vi "Main FPGA 5-axis for XYZ.vi"() -> ()   [LabVIEW 2014]
uses:
  <vilib>/Motion/MotorControl/_s/nism.interpretControlRegister.stateTransition.ctl
  <vilib>/Platform/TimedLoop/XDataNode/timing_clust.ctl
  <vilib>/Platform/TimedLoop/XDataNode/nitl_modes.ctl
  <vilib>/Platform/TimedLoop/XDataNode/wakeup.ctl
  <vilib>/Motion/MotorControl/_s/nism.digitalInputs.portA.ctl
  <vilib>/rvi/Emulation/niFpgaGetClockAttributes.vi
  <vilib>/rvi/Emulation/niFpgaSctlEmulationGetInTimedLoop.vi
  <vilib>/rvi/Emulation/niFpgaEmulationReportErrorSimple.vi
  Global FPGA.vi
  <vilib>/Motion/MotorControl/_s/nism.interpretControlRegister.indexed.vi
  <vilib>/rvi/Emulation/niFpgaProcessEmulError.vi
  <vilib>/Motion/MotorControl/_s/nism.mdo.read.positionLoopSyncData.vi
  <vilib>/Motion/MotorControl/_s/nism.mdo.read.splineData.vi
  <vilib>/Motion/MotorControl/_s/nism.generateStatusRegister.indexed.vi
  <vilib>/rvi/eio/common/nirviEmuTemplateMethod_errors.vi
  <vilib>/rvi/Emulation/niFpgaCriticalErrorInLSC.vi
  <vilib>/Motion/MotorControl/_s/nism.splineInterpolation.fxp.3.index.vi
  <vilib>/Motion/MotorControl/_s/nism.mdo.handler.indexed.vi
  <vilib>/Motion/MotorControl/_s/nism.digitalFilter.indexed.vi
  <vilib>/Motion/MotorControl/_s/nism.interpretDIOControl.portA.multiple.vi
  <vilib>/Motion/MotorControl/_s/nism.generateDIOStatus.portA.indexed.2.vi
  <vilib>/Motion/SoftMotion/Synchronization/nism.rioScan.generateSyncScan.vi
  <vilib>/eio/EIONode/EIONode.xnode
  <vilib>/Platform/TimedLoop/XDataNode/XDataNode.xnode
  <vilib>/Motion/MotorControl/NI_SoftMotion_MotorControlIP.lvlib
  <vilib>/Platform/TimedLoop/XDataNode/XDNodeRunTimeDep.lvlib
  <vilib>/Motion/SoftMotion/Synchronization/NI_SoftMotion_Synchronization.lvlib
panel:
  in  "Mod3/DIO31":bool
  in  "Mod3/DIO30":bool
  in  "Mod3/DIO29":bool
  in  "Mod3/DIO28":bool
  in  "Fwd 5":bool
  in  "Fwd 4":bool
  in  "Rev 5":bool
  in  "Rev 4":bool
  in  "Home 5":bool
  in  "Home 4":bool
  out "Home Limits":bool[](array[boolean])
  out "Fwd Limits":bool[](array[boolean])
  out "Rev Limits":bool[](array[boolean])
  out "Axis Positions":fxp<+/-,64,32>[](array[numeric])
  in  "STEP or CW? (T=STEP)":bool
  out "Drive Enable":bool[](array[boolean])
  in  "Enable Watchdog":bool
  in  "Pet Watchdog":bool
  in  "Watchdog Timeout Period (ticks)":u64=40000000 format="%.0p"
  out "Watchdog Timed Out?":bool
  out "Time Since Last Pet":u64
  in  "Enable value":bool
  in  "Drive Enable override?":bool
  out "State":T1=enum."Start --> Initializing" caption="state transition"
  in  "Sync Value":bool
  in  "Sync Enable override?":bool
  in  "Invert direction?":bool
  out "Sync is Fault":bool
  out "Sync is Locked":bool
  in  "minimum pulse":u16=40
  # "Synchronization Loop"
  # "Control Status Loop"
  # "Notes: \n1. This VI provides the communication interface between the NI SoftMotion Engine and the LabVIEW FPGA Module. You must compile this VI for a specific FPGA target before use. After compiling, run the VI before running any of the Express VI examples. For information on moving this example to another FPGA target, refer to ni.com/info and enter info code fpgaex.\n\n2. Only use the Reset Axis button if you are unable to communicate with the axis by any other means. This button resets the device state machine and other VIs to a known state. After resetting the axis, switch the NI Scan Engine from Active Mode to Configuration Mode, then back to Active Mode, before attempting to enable the axis."
  # "(These two buttons \nare for testing\npurposes.)"
  # "(These two buttons \nare for testing\npurposes.)"
  # "Step/Direction Loop"
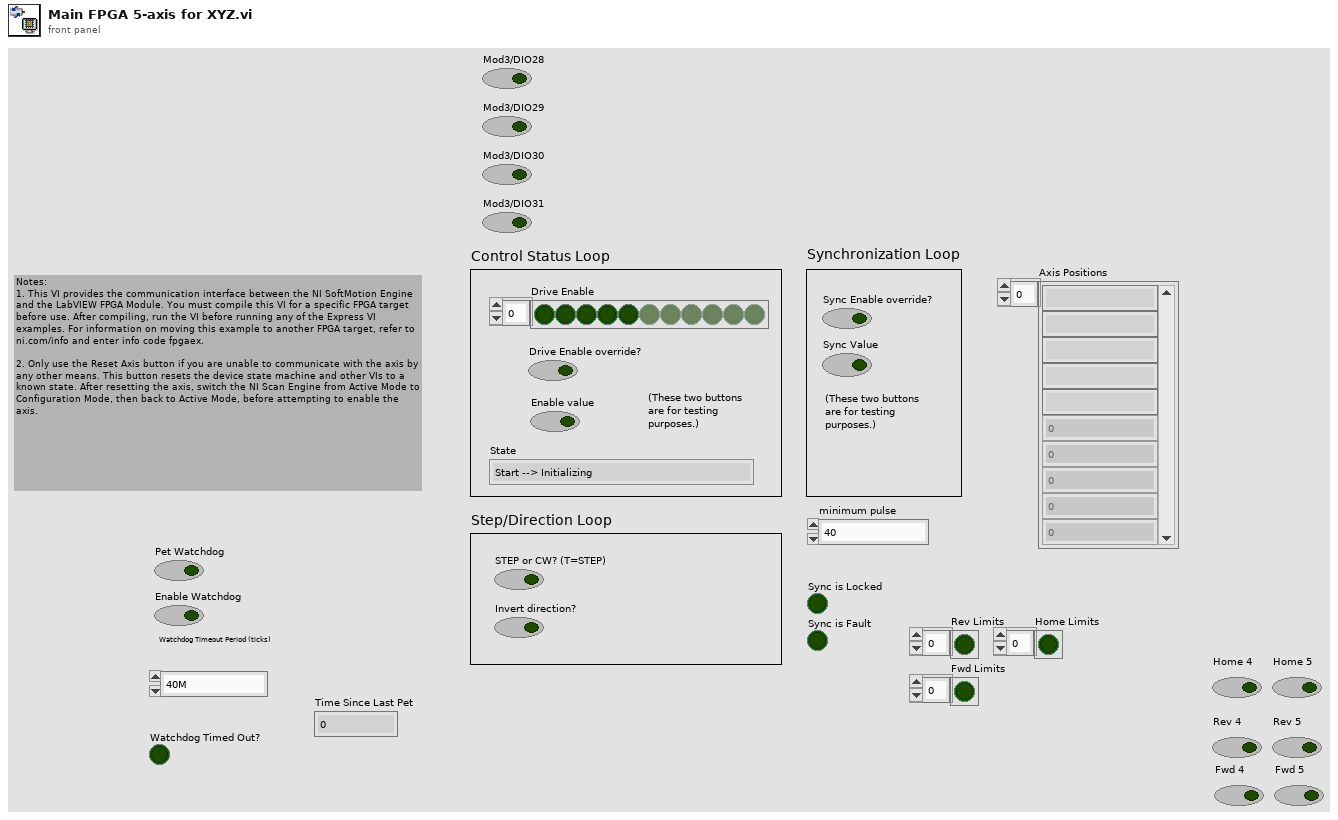
[diagram p1: front panel]
types:
  T1 = typedef "NI_SoftMotion_MotorControlIP.lvlib/nism.interpretControlRegister.stateTransition.ctl" = enum8{"Invalid", "Start --> Initializing", "Initializing --> Disabled", "Disabled --> Ready To Switch On", "Ready To Switch On --> Switched On", "Ready To Switch On --> Disable", "Switched On --> Operation Enable", "Switched On --> Ready To Switch On", "Switched On --> Disabled", "Operation Enable --> Switched On", "Operation Enable --> Ready To Switch On", "Operation Enable --> Disabled", "Fault --> Disabled", "Any --> Fault", "None"}
  T2 = typedef "NI_SoftMotion_Synchronization.lvlib/nism.softmotionScan.timerConfig.ctl" = cluster{"target period (clocks)":u16, "host period / target period":u16}
  T3 = typedef "NI_SoftMotion_MotorControlIP.lvlib/nism.mdo.splineData.ctl" = cluster{"spline type":T4, "traj per/spline per":u16, "spline per/traj per":fxp<+,32,0>}
  T4 = typedef "NI_SoftMotion_MotorControlIP.lvlib/nism.splineInterpolation.type.ctl" = u16
  T5 = typedef "XDNodeRunTimeDep.lvlib/timing_clust.ctl" = cluster{"Expected End [f-1]":u64, "Actual End [f-1]":u64, "Finished Late? [f-1]":bool, "Expected End [i-1]":u64, "Actual End [i-1]":u64, "Finished Late? [i-1]":bool, "Expected Start [i]":u64, "Actual Start [i]":u64, "Expected Start [f]":u64, "Actual Start [f]":u64, "Source Name":string, "Structure Name":string, "Period":i64, "Deadline":i64, "Offset":i64, "Start":i64, "Priority":i32, "Timeout":i32, "Mode":T6, "Wakeup Reason":T7, "Error":errorcluster, "Source Type":string, "Secondary Source Type":string, "Global End Time":u64, "Global Start Time":u64, "Frame Duration":u64, "Iteration Duration":u64, "Assigned CPU":i32, "I/O Scan Engine Mode":u32}
  T6 = typedef "XDNodeRunTimeDep.lvlib/nitl_modes.ctl" = enum32{"No Change", "Process missed periods, maintain original phase", "Discard missed periods, maintain original phase", "Process missed periods, ignore original phase", "Discard missed periods, ignore original phase"}
  T7 = typedef "XDNodeRunTimeDep.lvlib/wakeup.ctl" = enum32{"Normal", "Aborted", "Asynchronous wakeup", "Timing source error", "Timed loop error", "Timeout"}
  T8 = typedef "NI_SoftMotion_Synchronization.lvlib/nism.softmotionScan.timerControl.ctl" = cluster{"sm scan":bool, "sm scan count":u32, "sm scan enabled":bool}
  T9 = typedef "NI_SoftMotion_MotorControlIP.lvlib/nism.digitalInputs.portA.ctl" = cluster{"reverse limit":bool, "forward limit":bool, "home switch":bool, "digital input 0":bool, "digital input 1":bool, "digital input 2":bool, "digital input 3":bool}
  T10 = typedef "NI_SoftMotion_MotorControlIP.lvlib/nism.dio.portA.config.2.ctl" = cluster{"digital filter (us)":u16[], "safe state":T11[]}
  T11 = typedef "nism.safeStates.ctl" = enum8{"Low", "High", "No Change"}
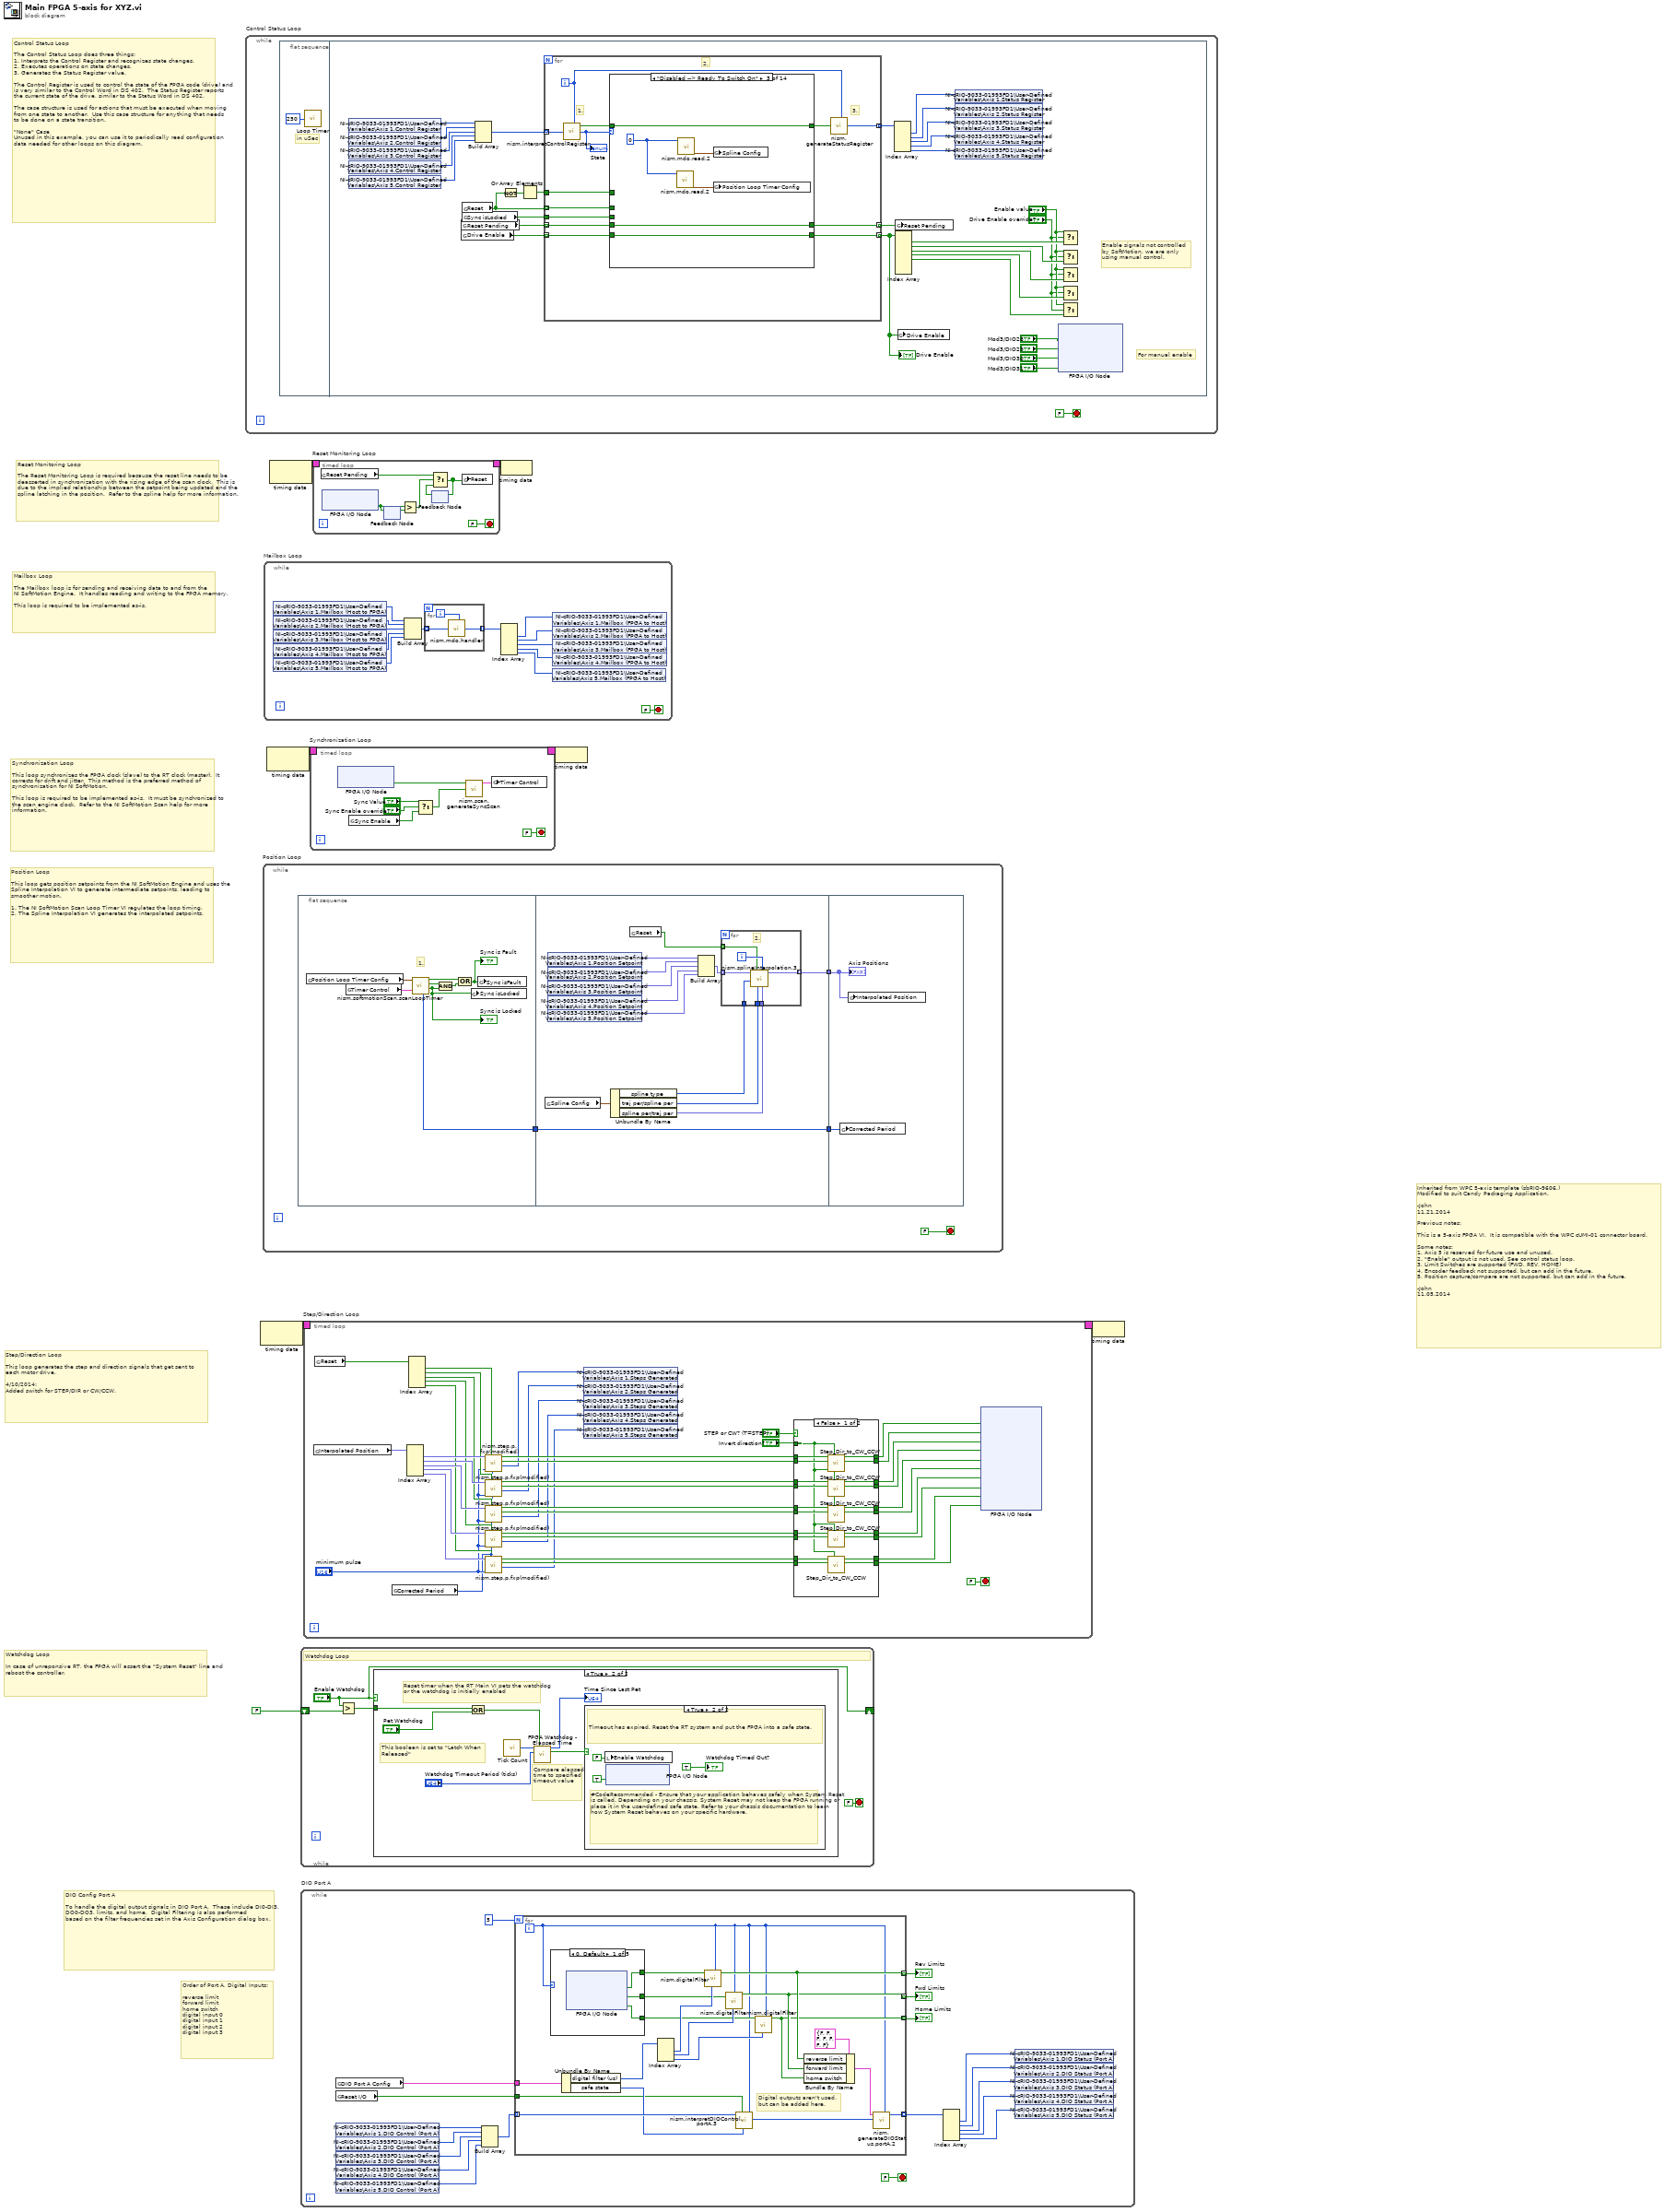
[diagram p0: block diagram]
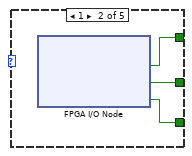
[diagram p2: hidden frame]
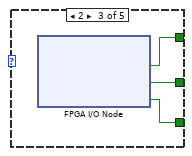
[diagram p3: hidden frame]
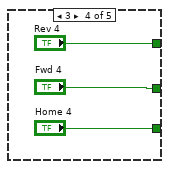
[diagram p4: hidden frame]
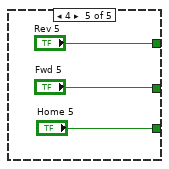
[diagram p5: hidden frame]
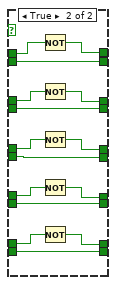
[diagram p9: hidden frame]
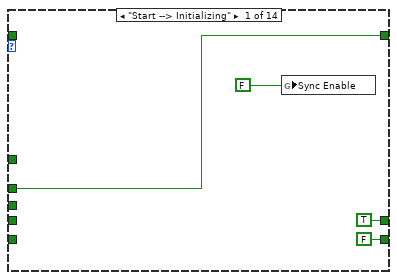
[diagram p10: hidden frame]
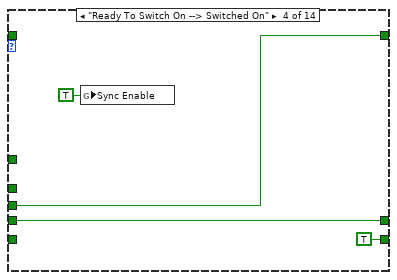
[diagram p12: hidden frame]
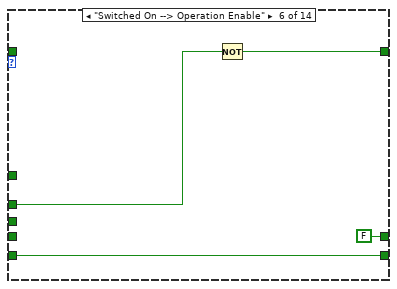
[diagram p14: hidden frame]
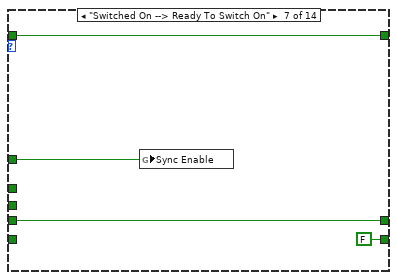
[diagram p15: hidden frame]
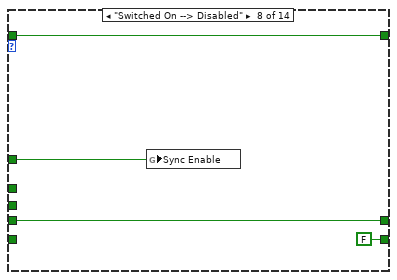
[diagram p16: hidden frame]
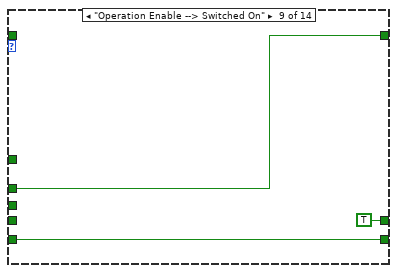
[diagram p17: hidden frame]
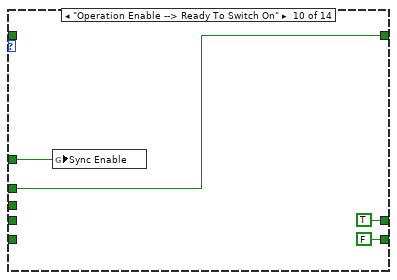
[diagram p18: hidden frame]
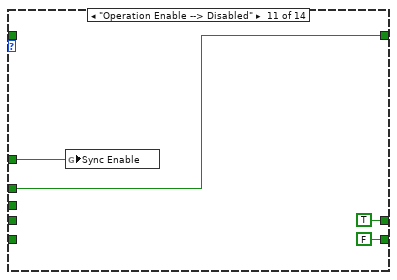
[diagram p19: hidden frame]
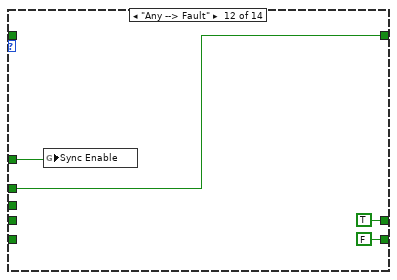
[diagram p20: hidden frame]
diagram:
  # "Inherited from WPC 5-axis template (sbRIO-9606.)\nModified to suit Candy Packaging Application.\n\n-John\n11.21.2014\n\nPrevious notes:\n\nThis is a 5-axis FPGA VI.  It is compatible with the WPC cUMI-01 connector board.\n\nSome notes:\n1. Axis 5 is reserved for future use and unused.\n2. \"Enable\" output is not used. See control status loop.\n3. Limit Switches are supported (FWD, REV, HOME)\n4. Encoder feedback not supported, but can add in the future.\n5. Position capture/compare are not supported, but can add in the future.\n\n-John\n11.05.2014"
  # "DIO Config Port A\n\nTo handle the digital output signals in DIO Port A.  These include DI0-DI3, DO0-DO3, limits, and home.  Digital Filtering is also performed\nbased on the filter frequencies set in the Axis Configuration dialog box."
  # "Order of Port A, Digital Inputs:\n\nreverse limit\nforward limit\nhome switch\ndigital input 0\ndigital input 1\ndigital input 2\ndigital input 3"
  # "Watchdog Loop\n\nIn case of unreponsive RT, the FPGA will assert the \"System Reset\" line and reboot the controller."
  # "Step/Direction Loop\n\nThis loop generates the step and direction signals that get sent to \neach motor drive.\n\n4/10/2014:\nAdded switch for STEP/DIR or CW/CCW."
  # "Position Loop\n\nThis loop gets position setpoints from the NI SoftMotion Engine and uses the Spline Interpolation VI to generate intermediate setpoints, leading to smoother motion.\n\n1. The NI SoftMotion Scan Loop Timer VI regulates the loop timing. \n2. The Spline Interpolation VI generates the interpolated setpoints."
  # "Synchronization Loop\n\nThis loop synchronizes the FPGA clock (slave) to the RT clock (master).  It corrects for drift and jitter.  This method is the preferred method of synchronization for NI SoftMotion.\n\nThis loop is required to be implemented as-is.  It must be synchronized to the scan engine clock.  Refer to the NI SoftMotion Scan help for more information."
  # "Mailbox Loop\n\nThe Mailbox loop is for sending and receiving data to and from the \nNI SoftMotion Engine.  It handles reading and writing to the FPGA memory.\n\nThis loop is required to be implemented as-is."
  # "Reset Monitoring Loop\n\nThe Reset Monitoring Loop is required because the reset line needs to be deasserted in synchronization with the rising edge of the scan clock.  This is due to the implied relationship between the setpoint being updated and the spline latching in the position.  Refer to the spline help for more information."
  # "Control Status Loop\n\nThe Control Status Loop does three things:\n1. Interprets the Control Register and recognizes state changes.\n2. Executes operations on state changes.\n3. Generates the Status Register value.\n\nThe Control Register is used to control the state of the FPGA code (drive) and is very similar to the Control Word in DS 402.  The Status Register reports the current state of the drive, similar to the Status Word in DS 402.\n\nThe case structure is used for actions that must be executed when moving from one state to another.  Use this case structure for anything that needs to be done on a state transition.\n\n\"None\" Case\nUnused in this example, you can use it to periodically read configuration data needed for other loops on this diagram."
  n1 = while "Control Status Loop" {
    stop <- FALSE stop-if-true
    n2 = flat-sequence {
      frame #0 {
        # "in uSec"
        n3 = call "Loop Timer"("Count(uSec)"=u32 250) -> ()  [unwired: 1 out]
      }
      frame #1 {
        # "For manual enable"
        # "Enable signals not controlled\nby SoftMotion, we are only\nusing manual control."
        n4 = shared-variable "NI-cRIO-9033-01993FD1\\User-Defined Variables\\Axis 1.Control Register"() -> (w30:u32)  [unwired: 1 in, 1 out]
        n5 = shared-variable "NI-cRIO-9033-01993FD1\\User-Defined Variables\\Axis 2.Control Register"() -> (w29:u32)  [unwired: 1 in, 1 out]
        n6 = shared-variable "NI-cRIO-9033-01993FD1\\User-Defined Variables\\Axis 3.Control Register"() -> (w28:u32)  [unwired: 1 in, 1 out]
        n7 = shared-variable "NI-cRIO-9033-01993FD1\\User-Defined Variables\\Axis 4.Control Register"() -> (w27:u32)  [unwired: 1 in, 1 out]
        n8 = shared-variable "NI-cRIO-9033-01993FD1\\User-Defined Variables\\Axis 5.Control Register"() -> (w26:u32)  [unwired: 1 in, 1 out]
        n9 = global read "Global FPGA.vi" "Reset Pending"() -> (w34:bool[])
        n10 = global read "Global FPGA.vi" "Drive Enable"() -> (w33:bool[])
        n11 = global read "Global FPGA.vi" "Reset"() -> (w35:bool[])
        n12 = global read "Global FPGA.vi" "Sync isLocked"() -> (w40:bool)
        n13 = Build Array(w30, w29, w28, w27, w26) -> (w39:u32[])
        n14 = Not(x=w35) -> (.not. x?=w37:bool[])
        n15 = Or Array Elements(Boolean array=w37) -> (logical OR=w36:bool)
        n16 = for {
          tunnel: w35 -> [w48] mode=indexing
          tunnel: w40 -> [w47]
          tunnel: w39 -> [w49] mode=indexing
          tunnel: [w46] -> w31 mode=indexing
          tunnel: [w45] -> w38 mode=indexing
          tunnel: [w44] -> w32 mode=indexing
          tunnel: w36 -> [w43]
          tunnel: w34 -> [w42] mode=indexing
          tunnel: w33 -> [w41] mode=indexing
          i -> [w50]
          # "3."
          # "2."
          # "1."
          n17 = call-poly <vilib>:"nism.interpretControlRegister.vi"("control register"=w49, "axis index"=w50) -> ("transition occurred"=w51:bool, "state transition"=w52:T1)  [unwired: 6 in]
          "State" <- w52
          n18 = case shown="\"Disabled --> Ready To Switch On\"" w52 {
            tunnel: w51 -> [_ w60 w66 _ w73 _ w81 w85 _ _ _ _ w105 _]
            tunnel: [w57 w60 w66 w68 w73 w77 w81 w85 w87 w90 w94 w98 w104 _] -> w53
            tunnel: w48 -> [w57 _ _ _ _ w76 _ _ w87 w90 w94 w98 _ _]
            tunnel: w47 -> [_ _ _ w68 _ _ _ _ _ _ _ _ _ _]
            tunnel: [TRUE ("Write.Reset Pending") w59 w63 w67 w72 FALSE ("Write.Reset Pending") w78 w82 TRUE ("Write.Reset Pending") TRUE ("Write.Reset Pending") TRUE ("Write.Reset Pending") TRUE ("Write.Reset Pending") w102 w107] -> w45
            tunnel: [FALSE ("Write.Drive Enable") w58 w62 TRUE ("Write.Drive Enable") w71 w74 FALSE ("Write.Drive Enable") FALSE ("Write.Drive Enable") w86 FALSE ("Write.Drive Enable") FALSE ("Write.Drive Enable") FALSE ("Write.Drive Enable") w101 w106] -> w44
            tunnel: w43 -> [_ _ _ _ _ _ w79 w83 _ w89 w93 w97 w103 _]
            tunnel: w42 -> [_ w59 w63 w67 w72 _ w78 w82 _ _ _ _ w102 w107]
            tunnel: w41 -> [_ w58 w62 _ w71 w74 _ _ w86 _ _ _ w101 w106]
            frame "Start --> Initializing" {
              n19 = global write "Global FPGA.vi" "Sync Enable"(FALSE ("Sync Enable")) -> ()
            }
            frame "Initializing --> Disabled" {
            }
            frame "Disabled --> Ready To Switch On" {
              w61 = 0 ("axis index")
              n20 = call-poly <vilib>:"nism.mdo.read.2.vi"("axis index"=w61) -> ("position loop sync"=w64:T2)  [unwired: 10 in]
              n21 = call-poly <vilib>:"nism.mdo.read.2.vi"("axis index"=w61) -> ("spline"=w65:T3)  [unwired: 10 in]
              n22 = global write "Global FPGA.vi" "Spline Config"(w65) -> ()
              n23 = global write "Global FPGA.vi" "Position Loop Timer Config"(w64) -> ()
            }
            frame "Ready To Switch On --> Switched On" {
              n24 = global write "Global FPGA.vi" "Sync Enable"(TRUE ("Sync Enable")) -> ()
            }
            frame "Ready To Switch On --> Disable" {
            }
            frame "Switched On --> Operation Enable" {
              n25 = Not(x=w76) -> (.not. x?=w77:bool)
            }
            frame "Switched On --> Ready To Switch On" {
              n26 = global write "Global FPGA.vi" "Sync Enable"(w79) -> ()
            }
            frame "Switched On --> Disabled" {
              n27 = global write "Global FPGA.vi" "Sync Enable"(w83) -> ()
            }
            frame "Operation Enable --> Switched On" {
            }
            frame "Operation Enable --> Ready To Switch On" {
              n28 = global write "Global FPGA.vi" "Sync Enable"(w89) -> ()
            }
            frame "Operation Enable --> Disabled" {
              n29 = global write "Global FPGA.vi" "Sync Enable"(w93) -> ()
            }
            frame "Any --> Fault" {
              n30 = global write "Global FPGA.vi" "Sync Enable"(w97) -> ()
            }
            frame "Fault --> Disabled" {
              # "wait one cycle for clear faults to have taken effect"
              n31 = global write "Global FPGA.vi" "Sync Enable"(w103) -> ()
              n32 = Not(x=w105) -> (.not. x?=w104:bool)
            }
            frame "None", Default {
            }
          }
          n33 = call-poly <vilib>:"nism.generateStatusRegister.vi"("transition success"=w53, "axis index"=w50) -> ("status register"=w46:u32)  [unwired: 7 in]
        }
        "Drive Enable" <- w32
        n34 = Index Array(array=w31) -> (element #1=w25:u32, element #2=w24:u32, element #3=w23:u32, element #4=w22:u32, element #5=w21:u32)  [unwired: 5 in]
        n35 = global write "Global FPGA.vi" "Reset Pending"(w38) -> ()
        n36 = Index Array(array=w32) -> (element #1=w20:bool, element #2=w19:bool, element #3=w18:bool, element #4=w17:bool, element #5=w16:bool)  [unwired: 8 in, 3 out]
        n37 = global write "Global FPGA.vi" "Drive Enable"(w32) -> ()
        n38 = shared-variable "NI-cRIO-9033-01993FD1\\User-Defined Variables\\Axis 1.Status Register"(w25) -> ()  [unwired: 1 in, 1 out]
        n39 = shared-variable "NI-cRIO-9033-01993FD1\\User-Defined Variables\\Axis 2.Status Register"(w24) -> ()  [unwired: 1 in, 1 out]
        n40 = shared-variable "NI-cRIO-9033-01993FD1\\User-Defined Variables\\Axis 3.Status Register"(w23) -> ()  [unwired: 1 in, 1 out]
        n41 = shared-variable "NI-cRIO-9033-01993FD1\\User-Defined Variables\\Axis 4.Status Register"(w22) -> ()  [unwired: 1 in, 1 out]
        n42 = shared-variable "NI-cRIO-9033-01993FD1\\User-Defined Variables\\Axis 5.Status Register"(w21) -> ()  [unwired: 1 in, 1 out]
        n43 = xnode "FPGA I/O Node"("Mod3/DIO28"="Mod3/DIO28", "Mod3/DIO29"="Mod3/DIO29", "Mod3/DIO30"="Mod3/DIO30", "Mod3/DIO31"="Mod3/DIO31") -> ()  [unwired: 4 in, 4 out]
        n44 = Select(t="Enable value", s="Drive Enable override?", f=w20) -> ()  [unwired: 1 out]
        n45 = Select(t="Enable value", s="Drive Enable override?", f=w19) -> ()  [unwired: 1 out]
        n46 = Select(t="Enable value", s="Drive Enable override?", f=w18) -> ()  [unwired: 1 out]
        n47 = Select(t="Enable value", s="Drive Enable override?", f=w17) -> ()  [unwired: 1 out]
        n48 = Select(t="Enable value", s="Drive Enable override?", f=w16) -> ()  [unwired: 1 out]
      }
    }
  }
  n49 = node-c288() -> (w7:T5)  [unwired: 1 in]
  n50 = while "Position Loop" {
    stop <- FALSE stop-if-true
    n51 = flat-sequence {
      tunnel: [w112] -> w108
      tunnel: [w126] -> w110
      tunnel: [w125] -> w109
      tunnel: w108 -> [w125]
      tunnel: w110 -> [w140]
      tunnel: w109 -> [w141]
      frame #0 {
        # "1."
        n52 = global read "Global FPGA.vi" "Position Loop Timer Config"() -> (w114:T2)
        n53 = global read "Global FPGA.vi" "Timer Control"() -> (w113:T8)
        n54 = call <vilib>:"nism.softmotionScan.scanLoopTimer.vi"("timer control"=w113, "timer config"=w114) -> ("scan running?"=w116:bool, "finished late?"=w118:bool, "fault occurred?"=w119:bool, "corrected period"=w112:u16)  [unwired: 5 in, 1 out]
        "Sync is Locked" <- w116
        n55 = Compound Arithmetic op=AND(w118, w116) -> (w117:bool)
        n56 = Compound Arithmetic op=OR(w119, w117) -> (w115:bool)
        "Sync is Fault" <- w115
        n57 = global write "Global FPGA.vi" "Sync isLocked"(w116) -> ()
        n58 = global write "Global FPGA.vi" "Sync isFault"(w115) -> ()
      }
      frame #1 {
        n59 = global read "Global FPGA.vi" "Spline Config"() -> (w128:T3)
        n60 = shared-variable "NI-cRIO-9033-01993FD1\\User-Defined Variables\\Axis 1.Position Setpoint"() -> (w124:fxp<+/-,64,32>)  [unwired: 1 in, 1 out]
        n61 = shared-variable "NI-cRIO-9033-01993FD1\\User-Defined Variables\\Axis 2.Position Setpoint"() -> (w123:fxp<+/-,64,32>)  [unwired: 1 in, 1 out]
        n62 = shared-variable "NI-cRIO-9033-01993FD1\\User-Defined Variables\\Axis 3.Position Setpoint"() -> (w122:fxp<+/-,64,32>)  [unwired: 1 in, 1 out]
        n63 = shared-variable "NI-cRIO-9033-01993FD1\\User-Defined Variables\\Axis 4.Position Setpoint"() -> (w121:fxp<+/-,64,32>)  [unwired: 1 in, 1 out]
        n64 = shared-variable "NI-cRIO-9033-01993FD1\\User-Defined Variables\\Axis 5.Position Setpoint"() -> (w120:fxp<+/-,64,32>)  [unwired: 1 in, 1 out]
        n65 = Unbundle By Name(w128) -> ("spline type"=w132:T4, "traj per/spline per"=w131:u16, "spline per/traj per"=w130:fxp<+,32,0>)
        n66 = global read "Global FPGA.vi" "Reset"() -> (w127:bool[])
        n67 = Build Array(w124, w123, w122, w121, w120) -> (w129:fxp<+/-,64,32>[])
        n68 = for {
          tunnel: w132 -> [w139]
          tunnel: w131 -> [w138]
          tunnel: w130 -> [w137]
          tunnel: w127 -> [w134] mode=indexing
          tunnel: w129 -> [w136] mode=indexing
          tunnel: [w133] -> w126 mode=indexing
          i -> [w135]
          # "2."
          n69 = call-poly <vilib>:"nism.splineInterpolation.3.vi"("1 / calls per sample"=w137, "index"=w135, "calls per sample"=w138, "reset"=w134, "spline type"=w139, "x"=w136) -> ("xi"=w133:fxp<+/-,64,32>)  [unwired: 4 in, 1 out]
        }
      }
      frame #2 {
        n70 = global write "Global FPGA.vi" "Corrected Period"(w141) -> ()
        n71 = global write "Global FPGA.vi" "Interpolated Position"(w140) -> ()
        "Axis Positions" <- w140
      }
    }
  }
  n72 = while "Mailbox Loop" {
    stop <- FALSE stop-if-true
    n73 = shared-variable "NI-cRIO-9033-01993FD1\\User-Defined Variables\\Axis 1.Mailbox (Host to FPGA)"() -> (w151:u64)  [unwired: 1 in, 1 out]
    n74 = shared-variable "NI-cRIO-9033-01993FD1\\User-Defined Variables\\Axis 2.Mailbox (Host to FPGA)"() -> (w150:u64)  [unwired: 1 in, 1 out]
    n75 = shared-variable "NI-cRIO-9033-01993FD1\\User-Defined Variables\\Axis 3.Mailbox (Host to FPGA)"() -> (w149:u64)  [unwired: 1 in, 1 out]
    n76 = shared-variable "NI-cRIO-9033-01993FD1\\User-Defined Variables\\Axis 4.Mailbox (Host to FPGA)"() -> (w148:u64)  [unwired: 1 in, 1 out]
    n77 = shared-variable "NI-cRIO-9033-01993FD1\\User-Defined Variables\\Axis 5.Mailbox (Host to FPGA)"() -> (w147:u64)  [unwired: 1 in, 1 out]
    n78 = Build Array(w151, w150, w149, w148, w147) -> (w153:u64[])
    n79 = for {
      tunnel: w153 -> [w157] mode=indexing
      tunnel: [w156] -> w152 mode=indexing
      i -> [w155]
      n80 = call-poly <vilib>:"nism.mdo.handler.vi"("mbox (host to fpga)"=w157, "axis index"=w155) -> ("mbox (fpga to host)"=w156:u64)  [unwired: 7 in]
    }
    n81 = Index Array(array=w152) -> (element #1=w146:u64, element #2=w145:u64, element #3=w144:u64, element #4=w143:u64, element #5=w142:u64)  [unwired: 5 in]
    n82 = shared-variable "NI-cRIO-9033-01993FD1\\User-Defined Variables\\Axis 5.Mailbox (FPGA to Host)"(w142) -> ()  [unwired: 1 in, 1 out]
    n83 = shared-variable "NI-cRIO-9033-01993FD1\\User-Defined Variables\\Axis 1.Mailbox (FPGA to Host)"(w146) -> ()  [unwired: 1 in, 1 out]
    n84 = shared-variable "NI-cRIO-9033-01993FD1\\User-Defined Variables\\Axis 2.Mailbox (FPGA to Host)"(w145) -> ()  [unwired: 1 in, 1 out]
    n85 = shared-variable "NI-cRIO-9033-01993FD1\\User-Defined Variables\\Axis 3.Mailbox (FPGA to Host)"(w144) -> ()  [unwired: 1 in, 1 out]
    n86 = shared-variable "NI-cRIO-9033-01993FD1\\User-Defined Variables\\Axis 4.Mailbox (FPGA to Host)"(w143) -> ()  [unwired: 1 in, 1 out]
  }
  n87 = node-c288() -> (w5:T5)  [unwired: 1 in]
  n88 = node-c288() -> (w3:T5)  [unwired: 1 in]
  n89 = while "RT Watchdog Loop" {
    shift-right: ["Enable Watchdog"] -> _
    shift-left: FALSE ("Enable RT Watchdog") -> [w161]
    stop <- FALSE stop-if-true
    # "Watchdog Loop"
    n90 = Greater?(x="Enable Watchdog", y=w161) -> (0:w158:bool)
    n91 = case shown="True" "Enable Watchdog" {
      tunnel: w158 -> [_ w164]
      frame False {
        # "This loop has to be explicitly enabled from the RT Main VI.  This reduces the possiblity of an endless reboot cycle."
      }
      frame True {
        # "This boolean is set to \"Latch When Released\""
        # "Compare elapsed time to specified timeout value"
        # "Reset timer when the RT Main VI pets the watchdog or the watchdog is initially enabled"
        n92 = Or(x=w164, y="Pet Watchdog") -> (x .or. y?=w163:bool)
        n93 = call "Tick Count"() -> ("Tick Count(Ticks)"=w167:u32)
        n94 = call "FPGA Watchdog - Elapsed Time.vi"("Reset"=w163, "Timeout Period"="Watchdog Timeout Period (ticks)", "Current Time"=w167) -> ("Timeout"=w162:bool, "Elapsed Time"=→"Time Since Last Pet":u64)  [unwired: 7 in]
        n95 = case shown="True" w162 {
          frame False {
            # "Timeout has not expired."
          }
          frame True {
            # "#CodeRecommended - Ensure that your application behaves safely when System Reset is called. Depending on your chassis, System Reset may not keep the FPGA running or place it in the user-defined safe state. Refer to your chassis documentation to learn how System Reset behaves on your specific hardware."
            # "Timeout has expired. Reset the RT system and put the FPGA into a safe state."
            n96 = local write "Enable Watchdog"(FALSE ("Enable RT Watchdog")) -> ()
            n97 = xnode "FPGA I/O Node"("System Reset"=TRUE ("RT Reset on Watchdog Failure?")) -> ()  [unwired: 1 in, 1 out]
            "Watchdog Timed Out?" <- TRUE ("Watchdog Timed Out?")
          }
        }
      }
    }
  }
  n98 = while "DIO Port A" {
    stop <- FALSE stop-if-true
    n99 = global read "Global FPGA.vi" "DIO Port A Config"() -> (w189:T10)
    n100 = global read "Global FPGA.vi" "Reset I/O"() -> (w188:bool)
    n101 = shared-variable "NI-cRIO-9033-01993FD1\\User-Defined Variables\\Axis 1.DIO Control (Port A)"() -> (w186:u32)  [unwired: 1 in, 1 out]
    n102 = shared-variable "NI-cRIO-9033-01993FD1\\User-Defined Variables\\Axis 2.DIO Control (Port A)"() -> (w185:u32)  [unwired: 1 in, 1 out]
    n103 = shared-variable "NI-cRIO-9033-01993FD1\\User-Defined Variables\\Axis 3.DIO Control (Port A)"() -> (w184:u32)  [unwired: 1 in, 1 out]
    n104 = shared-variable "NI-cRIO-9033-01993FD1\\User-Defined Variables\\Axis 4.DIO Control (Port A)"() -> (w183:u32)  [unwired: 1 in, 1 out]
    n105 = shared-variable "NI-cRIO-9033-01993FD1\\User-Defined Variables\\Axis 5.DIO Control (Port A)"() -> (w182:u32)  [unwired: 1 in, 1 out]
    n106 = Build Array(w186, w185, w184, w183, w182) -> (w181:u32[])
    n107 = for {
      N: 5 -> [_]
      tunnel: [w209] -> w175 mode=indexing
      tunnel: w181 -> [w208] mode=indexing
      tunnel: w189 -> [w206]
      tunnel: w188 -> [w204]
      tunnel: [w196] -> w174 mode=indexing
      tunnel: [w195] -> w173 mode=indexing
      tunnel: [w194] -> w172 mode=indexing
      i -> [w193]
      # "Digital outputs aren't used,\nbut can be added here."
      n108 = case shown="0, Default" w193 {
        tunnel: [w212 w215 w218 "Rev 4" "Rev 5"] -> w199
        tunnel: [w210 w213 w216 "Home 4" "Home 5"] -> w198
        tunnel: [w211 w214 w217 "Fwd 4" "Fwd 5"] -> w197
        frame 0, Default {
          n109 = xnode "FPGA I/O Node"() -> ("Mod3/DIO0"=w212:bool, "Mod3/DIO1"=w211:bool, "Mod3/DIO2"=w210:bool)  [unwired: 3 in, 3 out]
        }
        frame 1 {
          n110 = xnode "FPGA I/O Node"() -> ("Mod3/DIO3"=w215:bool, "Mod3/DIO4"=w214:bool, "Mod3/DIO5"=w213:bool)  [unwired: 3 in, 3 out]
        }
        frame 2 {
          n111 = xnode "FPGA I/O Node"() -> ("Mod3/DIO6"=w218:bool, "Mod3/DIO7"=w217:bool, "Mod3/DIO8"=w216:bool)  [unwired: 3 in, 3 out]
        }
        frame 3 {
        }
        frame 4 {
        }
      }
      n112 = Unbundle By Name(w206) -> ("digital filter (us)"=w200:u16[], "safe state"=w205:T11[])
      n113 = Index Array(array=w200) -> (element #1=w201:u16, element #2=w202:u16, element #3=w203:u16)  [unwired: 3 in]
      n114 = call-poly <vilib>:"nism.digitalFilter.vi"("index"=w193, "filter value (us)"=w201, "input signal"=w199) -> ("output signal"=w196:bool)  [unwired: 8 in]
      n115 = call-poly <vilib>:"nism.digitalFilter.vi"("index"=w193, "filter value (us)"=w202, "input signal"=w197) -> ("output signal"=w195:bool)  [unwired: 8 in]
      n116 = call-poly <vilib>:"nism.interpretDIOControl.portA.3.vi"("index"=w193, "safe state"=w205, "reset"=w204, "dio control(port a)"=w208) -> ("reset latches"=w191:u8)  [unwired: 6 in, 1 out]
      n117 = call-poly <vilib>:"nism.digitalFilter.vi"("index"=w193, "filter value (us)"=w203, "input signal"=w198) -> ("output signal"=w194:bool)  [unwired: 8 in]
      n118 = Bundle By Name(cluster=T9 {"reverse limit"=FALSE, "forward limit"=FALSE, "home switch"=FALSE, "digital input 0"=FALSE, "digital input 1"=FALSE, "digital input 2"=FALSE, "digital input 3"=FALSE} ("$(driveInterface.digitalInputs.shortName)"), "reverse limit"=w196, "forward limit"=w195, "home switch"=w194) -> (w192:T9)
      n119 = call-poly <vilib>:"nism.generateDIOStatus.portA.2.vi"("index"=w193, "reset latches"=w191, "digital inputs"=w192) -> ("dio status(port a)"=w209:u32)  [unwired: 8 in]
    }
    "Rev Limits" <- w174
    "Fwd Limits" <- w173
    "Home Limits" <- w172
    n120 = Index Array(array=w175) -> (element #1=w180:u32, element #2=w179:u32, element #3=w178:u32, element #4=w177:u32, element #5=w176:u32)  [unwired: 5 in]
    n121 = shared-variable "NI-cRIO-9033-01993FD1\\User-Defined Variables\\Axis 1.DIO Status (Port A)"(w180) -> ()  [unwired: 1 in, 1 out]
    n122 = shared-variable "NI-cRIO-9033-01993FD1\\User-Defined Variables\\Axis 2.DIO Status (Port A)"(w179) -> ()  [unwired: 1 in, 1 out]
    n123 = shared-variable "NI-cRIO-9033-01993FD1\\User-Defined Variables\\Axis 3.DIO Status (Port A)"(w178) -> ()  [unwired: 1 in, 1 out]
    n124 = shared-variable "NI-cRIO-9033-01993FD1\\User-Defined Variables\\Axis 4.DIO Status (Port A)"(w177) -> ()  [unwired: 1 in, 1 out]
    n125 = shared-variable "NI-cRIO-9033-01993FD1\\User-Defined Variables\\Axis 5.DIO Status (Port A)"(w176) -> ()  [unwired: 1 in, 1 out]
  }
  n126 = timed-loop "Step/Direction Loop" {
    timing: w7 -> [_]
    timing-out: [_] -> w6
    stop <- FALSE stop-if-true
    n127 = global read "Global FPGA.vi" "Interpolated Position"() -> (w265:fxp<+/-,64,32>[])
    n128 = global read "Global FPGA.vi" "Reset"() -> (w259:bool[])
    n129 = global read "Global FPGA.vi" "Corrected Period"() -> (w235:u16)
    n130 = Index Array(array=w265) -> (element #1=w264:fxp<+/-,64,32>, element #2=w263:fxp<+/-,64,32>, element #3=w262:fxp<+/-,64,32>, element #4=w261:fxp<+/-,64,32>, element #5=w260:fxp<+/-,64,32>)  [unwired: 5 in]
    n131 = Index Array(array=w259) -> (element #1=w258:bool, element #2=w257:bool, element #3=w256:bool, element #4=w255:bool, element #5=w254:bool)  [unwired: 5 in]
    n132 = call "nism.step.p.fxp(modified).vi"("calls per sample"=w235, "reset"=w258, "minimum pulse"="minimum pulse", "position setpoint"=w264) -> ("steps generated"=w240:i32, "step"=w252:bool, "direction"=w253:bool)  [unwired: 4 in, 1 out]
    n133 = call "nism.step.p.fxp(modified).vi"("calls per sample"=w235, "reset"=w257, "minimum pulse"="minimum pulse", "position setpoint"=w263) -> ("steps generated"=w239:i32, "step"=w250:bool, "direction"=w251:bool)  [unwired: 4 in, 1 out]
    n134 = call "nism.step.p.fxp(modified).vi"("calls per sample"=w235, "reset"=w256, "minimum pulse"="minimum pulse", "position setpoint"=w262) -> ("steps generated"=w238:i32, "step"=w248:bool, "direction"=w249:bool)  [unwired: 4 in, 1 out]
    n135 = call "nism.step.p.fxp(modified).vi"("calls per sample"=w235, "reset"=w255, "minimum pulse"="minimum pulse", "position setpoint"=w261) -> ("steps generated"=w237:i32, "step"=w246:bool, "direction"=w247:bool)  [unwired: 4 in, 1 out]
    n136 = call "nism.step.p.fxp(modified).vi"("calls per sample"=w235, "reset"=w254, "minimum pulse"="minimum pulse", "position setpoint"=w260) -> ("steps generated"=w236:i32, "step"=w244:bool, "direction"=w245:bool)  [unwired: 4 in, 1 out]
    n137 = shared-variable "NI-cRIO-9033-01993FD1\\User-Defined Variables\\Axis 1.Steps Generated"(w240) -> ()  [unwired: 1 in, 1 out]
    n138 = shared-variable "NI-cRIO-9033-01993FD1\\User-Defined Variables\\Axis 2.Steps Generated"(w239) -> ()  [unwired: 1 in, 1 out]
    n139 = shared-variable "NI-cRIO-9033-01993FD1\\User-Defined Variables\\Axis 3.Steps Generated"(w238) -> ()  [unwired: 1 in, 1 out]
    n140 = shared-variable "NI-cRIO-9033-01993FD1\\User-Defined Variables\\Axis 4.Steps Generated"(w237) -> ()  [unwired: 1 in, 1 out]
    n141 = shared-variable "NI-cRIO-9033-01993FD1\\User-Defined Variables\\Axis 5.Steps Generated"(w236) -> ()  [unwired: 1 in, 1 out]
    n142 = case shown="False" "STEP or CW? (T=STEP)" {
      tunnel: w253 -> [w287 w307]
      tunnel: w252 -> [w286 w297]
      tunnel: w251 -> [w285 w305]
      tunnel: w250 -> [w284 w295]
      tunnel: w249 -> [w283 w303]
      tunnel: w248 -> [w282 w293]
      tunnel: w247 -> [w281 w301]
      tunnel: w246 -> [w280 w291]
      tunnel: w245 -> [w279 w299]
      tunnel: w244 -> [w278 w289]
      tunnel: "Invert direction?" -> [w267 w308]
      tunnel: [w277 w306] -> w234
      tunnel: [w276 w296] -> w233
      tunnel: [w275 w304] -> w232
      tunnel: [w274 w294] -> w231
      tunnel: [w273 w302] -> w230
      tunnel: [w272 w292] -> w229
      tunnel: [w271 w300] -> w228
      tunnel: [w270 w290] -> w227
      tunnel: [w269 w298] -> w225
      tunnel: [w268 w288] -> w226
      frame False {
        n143 = call "Step_Dir_to_CW_CCW.vi"("invert"=w267, "step"=w286, "direction"=w287) -> ("CCW"=w276:bool, "CW"=w277:bool)  [unwired: 7 in]
        n144 = call "Step_Dir_to_CW_CCW.vi"("invert"=w267, "step"=w284, "direction"=w285) -> ("CCW"=w274:bool, "CW"=w275:bool)  [unwired: 7 in]
        n145 = call "Step_Dir_to_CW_CCW.vi"("invert"=w267, "step"=w282, "direction"=w283) -> ("CCW"=w272:bool, "CW"=w273:bool)  [unwired: 7 in]
        n146 = call "Step_Dir_to_CW_CCW.vi"("invert"=w267, "step"=w280, "direction"=w281) -> ("CCW"=w270:bool, "CW"=w271:bool)  [unwired: 7 in]
        n147 = call "Step_Dir_to_CW_CCW.vi"("invert"=w267, "step"=w278, "direction"=w279) -> ("CCW"=w268:bool, "CW"=w269:bool)  [unwired: 7 in]
      }
      frame True {
        n148 = case shown="False" w308 {
          tunnel: w307 -> [w318 w333]
          tunnel: [w318 w332] -> w306
          tunnel: w305 -> [w316 w331]
          tunnel: [w316 w330] -> w304
          tunnel: w303 -> [w314 w329]
          tunnel: [w314 w328] -> w302
          tunnel: w301 -> [w312 w327]
          tunnel: [w312 w326] -> w300
          tunnel: w299 -> [w310 w325]
          tunnel: [w310 w324] -> w298
          tunnel: w297 -> [w317 w323]
          tunnel: [w317 w323] -> w296
          tunnel: w295 -> [w315 w322]
          tunnel: [w315 w322] -> w294
          tunnel: w293 -> [w313 w321]
          tunnel: [w313 w321] -> w292
          tunnel: w291 -> [w311 w320]
          tunnel: [w311 w320] -> w290
          tunnel: w289 -> [w309 w319]
          tunnel: [w309 w319] -> w288
          frame False {
          }
          frame True {
            n149 = Not(x=w333) -> (.not. x?=w332:bool)
            n150 = Not(x=w331) -> (.not. x?=w330:bool)
            n151 = Not(x=w329) -> (.not. x?=w328:bool)
            n152 = Not(x=w327) -> (.not. x?=w326:bool)
            n153 = Not(x=w325) -> (.not. x?=w324:bool)
          }
        }
      }
    }
    n154 = xnode "FPGA I/O Node"("Mod1/DIO0"=w234, "Mod1/DIO1"=w233, "Mod1/DIO2"=w232, "Mod1/DIO3"=w231, "Mod1/DIO4"=w230, "Mod1/DIO5"=w229, "Mod1/DIO6"=w228, "Mod1/DIO7"=w227, "Mod2/DIO0"=w225, "Mod2/DIO1"=w226) -> ()  [unwired: 10 in, 10 out]
  }
  n155 = timed-loop "Synchronization Loop" {
    timing: w5 -> [_]
    timing-out: [_] -> w4
    stop <- FALSE stop-if-true
    n156 = xnode "FPGA I/O Node"() -> ("Scan Clock"=w340:bool)  [unwired: 1 in, 1 out]
    n157 = global read "Global FPGA.vi" "Sync Enable"() -> (w339:bool)
    n158 = Select(t="Sync Value", s="Sync Enable override?", f=w339) -> (s? t:f=w336:bool)
    n159 = call-poly <vilib>:"nism.scan.generateSyncScan.vi"("scan enable?"=w336, "scan clock"=w340) -> ("timer control"=w341:T8)  [unwired: 3 in]
    n160 = global write "Global FPGA.vi" "Timer Control"(w341) -> ()
  }
  n161 = timed-loop "Reset Monitoring Loop" {
    timing: w3 -> [_]
    timing-out: [_] -> w2
    stop <- FALSE stop-if-true
    n162 = global read "Global FPGA.vi" "Reset Pending"() -> (w347:bool[])
    n163 = xnode "FPGA I/O Node"() -> ("Scan Clock"=w346:bool)  [unwired: 1 in, 1 out]
    n164 = feedback-in #1(w346) -> ()
    n165 = feedback #1() -> (w345:bool)  [unwired: 1 in]
    n166 = Greater?(x=w346, y=w345) -> (0:w351:bool)
    n167 = feedback #2() -> (w350:bool[])  [unwired: 1 in]
    n168 = Select(t=w347, s=w351, f=w350) -> (s? t:f=w348:bool[])
    n169 = feedback-in #2(w348) -> ()
    n170 = global write "Global FPGA.vi" "Reset"(w348) -> ()
  }
  n171 = node-c288(w2) -> ()
  n172 = node-c288(w4) -> ()
  n173 = node-c288(w6) -> ()
